vi "Write Last messages.vi"(8 "error in (no error)":errorcluster, 10 "Last messages":string[](array[string]), 11 "Header content in":refnum<class "Header content.lvclass">) -> (0 "error out":errorcluster, 3 "Header content out":refnum<class "Header content.lvclass">)   [LabVIEW 2018, in "Header content.lvclass"]
uses:
  Header content.lvclass
  Header content.lvclass/Header content.ctl
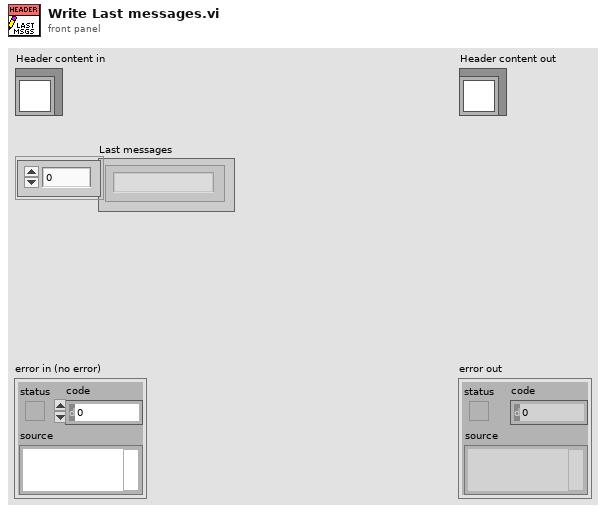
[diagram p1: front panel]
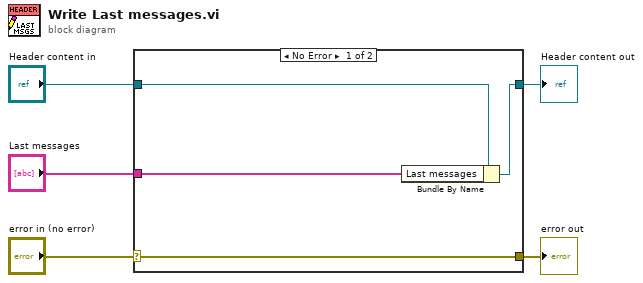
[diagram p0: block diagram]
diagram:
  n1 = case shown="No Error" "error in (no error)" {
    selector: "error in (no error)" -> [w9 w10]
    tunnel: [w9 w10] -> w4
    tunnel: [w7 w11] -> w2
    tunnel: "Header content in" -> [w8 w11]
    tunnel: "Last messages" -> [w6 _]
    frame No Error {
      n2 = Bundle By Name(cluster=w8, "Last messages"=w6) -> (w7:refnum<class "Header content.lvclass">)
    }
    frame Error {
    }
  }
  "error out" <- w4
  "Header content out" <- w2
